vi "Y=A’BC+AB’C’+AC using NAND GATES.vi"() -> ()   [LabVIEW 2018]
panel:
  in  "?":string
  in  "?":string
  out "Y":bool
  in  "C":bool
  in  "B":bool
  in  "A":bool
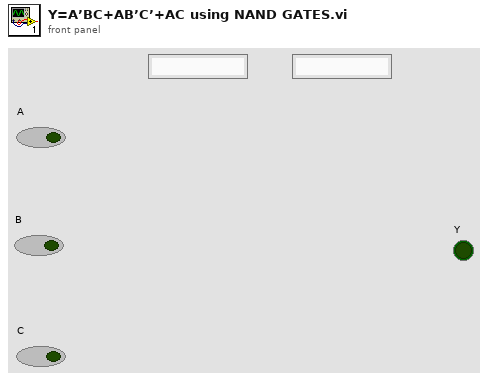
[diagram p1: front panel]
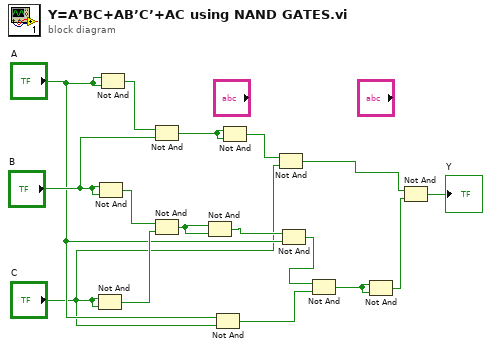
[diagram p0: block diagram]
diagram:
  n1 = Not And(1:"C", 2:"C") -> (0:w11:bool)
  n2 = Not And(1:"B", 2:"B") -> (0:w12:bool)
  n3 = Not And(1:"A", 2:"A") -> (0:w16:bool)
  n4 = Not And(1:"B", 2:w16) -> (0:w14:bool)
  n5 = Not And(1:w11, 2:w12) -> (0:w10:bool)
  n6 = Not And(1:w10, 2:w10) -> (0:w9:bool)
  n7 = Not And(1:"C", 2:"A") -> (0:w5:bool)
  n8 = Not And(1:w14, 2:w14) -> (0:w13:bool)
  n9 = Not And(1:"C", 2:w13) -> (0:w2:bool)
  n10 = Not And(1:"A", 2:w9) -> (0:w4:bool)
  n11 = Not And(1:w5, 2:w4) -> (0:w3:bool)
  n12 = Not And(1:w3, 2:w3) -> (0:w1:bool)
  n13 = Not And(1:w1, 2:w2) -> (0:→"Y":bool)
